vi "Fdx Write Frame to Tx Queue.vi"(6 "Frame Size":i32=-1, 8 "error in (no error)":errorcluster, 9 "Frame in":u8[](array[numeric]), 10 "HeaderInfo":T1={"InterFrameGap"=0, "PacketGroupWaitTime"=10000, "PayloadBufferMode"=0, "PayloadGenerationMode"=0, "PreambleCount"=7, "Skew"=0, "NetSelect"=4, "FrameStartMode"=1, "PhysErrorInjection"=0, "SequenceNumberInit"=65535, "SequenceNumberOffset"=65535} {"NetSelect" items=["FDX_TX_FRAME_DLY_A"=0, "FDX_TX_FRAME_DLY_B"=1, "FDX_TX_FRAME_BOTH "=3, "FDX_TX_FRAME_ONLY_A"=4, "FDX_TX_FRAME_ONLY_B "=5]; "FrameStartMode" items=["FDX_TX_FRAME_START_IFG", "FDX_TX_FRAME_START_PGWT", "FDX_TX_FRAME_START_TRG"]; "PhysErrorInjection" items=["FDX_TX_FRAME_ERR_OFF"=0, "FDX_TX_FRAME_ERR_CRC"=1, "FDX_TX_FRAME_ERR_ALI"=2, "FDX_TX_FRAME_ERR_PRE"=4, "FDX_TX_FRAME_ERR_PHY"=8]; "SequenceNumberInit" items=["FDX_TX_FRAME_SEQ_INIT_AUTO"=65535]; "SequenceNumberOffset" items=["FDX_TX_FRAME_SEQ_OFFS_AUTO "=65535]; "PayloadGenerationMode" items=["FDX_TX_FRAME_PGM_USER"=0, "FDX_TX_FRAME_PGM_IP_PART"=1, "FDX_TX_FRAME_PGM_IP_FULL"=2, "FDX_TX_FRAME_PGM_IP_PART_TT"=10, "FDX_TX_FRAME_PGM_IP_FULL_TT"=20]; "PayloadBufferMode" items=["FDX_TX_FRAME_PBM_STD", "FDX_TX_FRAME_PBM_MAC", "FDX_TX_FRAME_PBM_UDP"]}, 11 "InstrumentHandle_port in":u32) -> (0 "error out":errorcluster, 3 "InstrumentHandle_port out":u32)   [LabVIEW 2020, in "AIM664LV.lvlib"]
doc: "This function is used to write Entries to a Transmit Queue from a provided buffer. For this write function the number of Entries and the number of bytes to write needs to be specified. The entries will always be queued at the end of the transmit queue."
uses:
  AIM664LV.lvlib
  _controls/queue_header_generic.ctl
panel:
  out "bytesWritten":i32
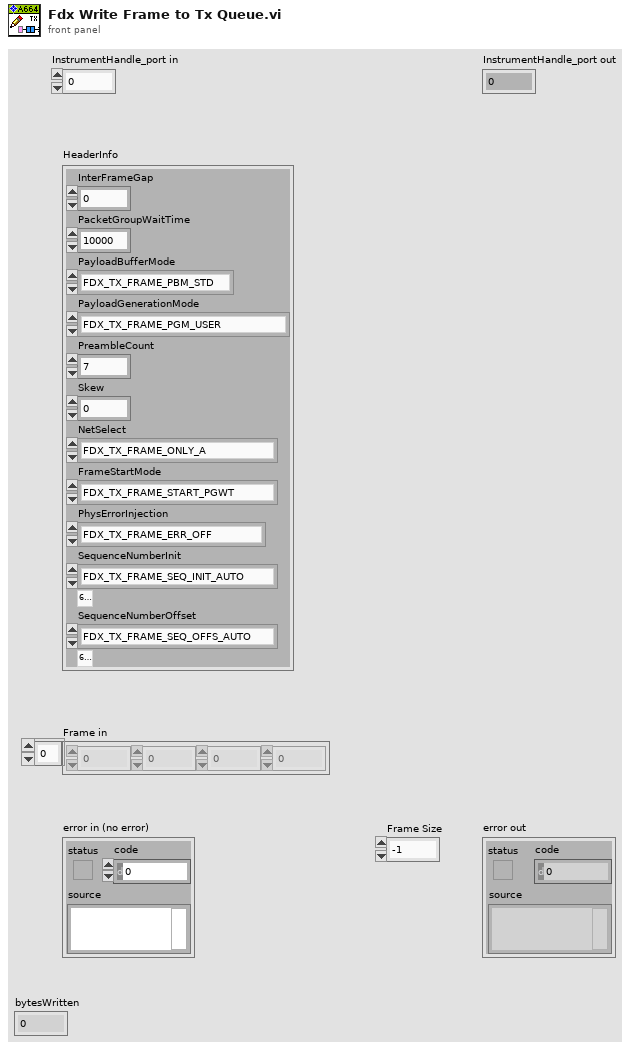
[diagram p1: front panel]
types:
  T1 = typedef "AIM664LV.lvlib/queue_header_generic.ctl" = cluster{"InterFrameGap":u32, "PacketGroupWaitTime":u32, "PayloadBufferMode":u8, "PayloadGenerationMode":u8, "PreambleCount":u8, "Skew":u32, "NetSelect":u8, "FrameStartMode":u8, "PhysErrorInjection":u32, "SequenceNumberInit":u16, "SequenceNumberOffset":u16}
  T2 = cluster{"HeaderType":u32, "EntryCount":u32, "WriteBytes":u32, "FrameSize":u16, "FrameType":u8, "InterFrameGap":u32, "PacketGroupWaitTime":u32, "PayloadBufferMode":u8, "PayloadGenerationMode":u8, "BufferQueueHandle":u32, "ExternalStrobe":u8, "PreambleCount":u8, "Skew":u32, "NetSelect":u8, "FrameStartMode":u8, "PhysErrorInjection":u32, "SequenceNumberInit":u16, "SequenceNumberOffset":u16, "Code":u8, "Interrupt":u8, "Data":u8[]}
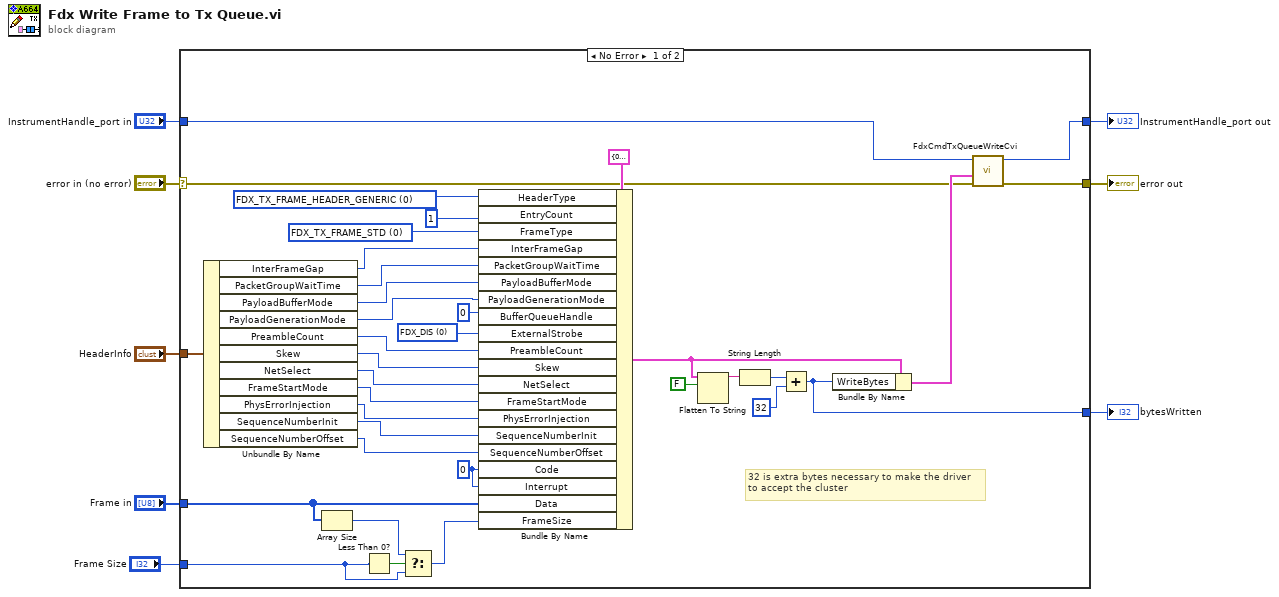
[diagram p0: block diagram]
diagram:
  n1 = case shown="No Error" "error in (no error)" {
    selector: "error in (no error)" -> [w17 w45]
    tunnel: "InstrumentHandle_port in" -> [w16 w44]
    tunnel: [w43 w45] -> w6
    tunnel: [w10 _] -> w5
    tunnel: "Frame in" -> [w23 _]
    tunnel: "HeaderInfo" -> [w33 _]
    tunnel: [w15 w44] -> w2
    tunnel: "Frame Size" -> [w13 _]
    frame No Error {
      w22 = u8 0 ("Code")
      w32 = u8 0 items=["FDX_DIS", "FDX_ENA"] ("ExternalStrobe")
      w34 = u8 0 items=["FDX_TX_FRAME_STD", "FDX_TX_FRAME_INSTR"] ("FrameType")
      w36 = u32 0 items=["FDX_TX_FRAME_HEADER_GENERIC ", "FDX_TX_FRAME_HEADER_REPLAY"] ("HeaderType")
      # "32 is extra bytes necessary to make the driver\nto accept the cluster"
      n2 = Unbundle By Name(w33) -> ("InterFrameGap"=w31:u32, "PacketGroupWaitTime"=w30:u32, "PayloadBufferMode"=w29:u8, "PayloadGenerationMode"=w28:u8, "PreambleCount"=w26:u8, "Skew"=w25:u32, "NetSelect"=w24:u8, "FrameStartMode"=w18:u8, "PhysErrorInjection"=w19:u32, "SequenceNumberInit"=w20:u16, "SequenceNumberOffset"=w21:u16)
      n3 = Array Size(array=w23) -> (size(s)=w12:i32)
      n4 = Less Than 0?(x=w13) -> (x < 0?=w14:bool)
      n5 = Select(t=w12, s=w14, f=w13) -> (s? t:f=w11:i32)
      n6 = Bundle By Name(cluster=T2 {"HeaderType"=0, "EntryCount"=0, "WriteBytes"=0, "FrameSize"=0, "FrameType"=0, "InterFrameGap"=0, "PacketGroupWaitTime"=0, "PayloadBufferMode"=0, "PayloadGenerationMode"=0, "BufferQueueHandle"=0, "ExternalStrobe"=0, "PreambleCount"=0, "Skew"=0, "NetSelect"=0, "FrameStartMode"=0, "PhysErrorInjection"=0, "SequenceNumberInit"=0, "SequenceNumberOffset"=0, "Code"=0, "Interrupt"=0, "Data"=[]} ("TxQueueWriteIn"), "HeaderType"=w36, "EntryCount"=u32 1, "FrameType"=w34, "InterFrameGap"=w31, "PacketGroupWaitTime"=w30, "PayloadBufferMode"=w29, "PayloadGenerationMode"=w28, "BufferQueueHandle"=u32 0, "ExternalStrobe"=w32, "PreambleCount"=w26, "Skew"=w25, "NetSelect"=w24, "FrameStartMode"=w18, "PhysErrorInjection"=w19, "SequenceNumberInit"=w20, "SequenceNumberOffset"=w21, "Code"=w22, "Interrupt"=w22, "Data"=w23, "FrameSize"=w11) -> (w39:T2)
      n7 = Flatten To String(anything=w39, prepend array or string size? (T)=FALSE) -> (data string=w41:string)  [unwired: 2 in, 2 out]
      n8 = String Length(string=w41) -> (length=w37:i32)
      n9 = Add(x=w37, y=32) -> (x+y=w10:i32)
      n10 = Bundle By Name(cluster=w39, "WriteBytes"=w10) -> (w38:T2)
      n11 = call "FdxCmdTxQueueWriteCvi.vi"("error in"=w17, "TxQueueWriteIn"=w38, "InstrumentHandle_port"=w16) -> ("error out"=w43:errorcluster, "InstrumentHandle_port"=w15:u32)  [unwired: 7 in]
    }
    frame Error {
    }
  }
  "error out" <- w6
  "InstrumentHandle_port out" <- w2
  "bytesWritten" <- w5
